vi "Host - Is FoE New.vi"(8 "error in (no error)":errorcluster, 10 "bitfile path in":path, 11 "Slave Ref in":refnum<k21>) -> (0 "error out":errorcluster, 3 "Slave Ref out":refnum<k21>)   [LabVIEW 2016, in "Scan Engine Custom Device.lvlib"]
uses:
  Scan Engine Custom Device.lvlib
  <resource>/objmgr/IndComECAT.rc
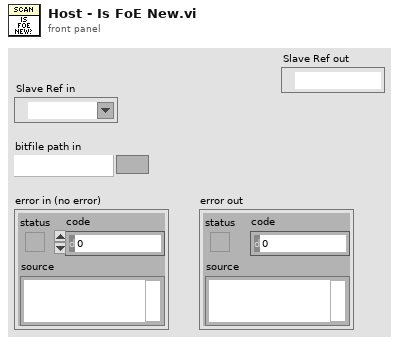
[diagram p1: front panel]
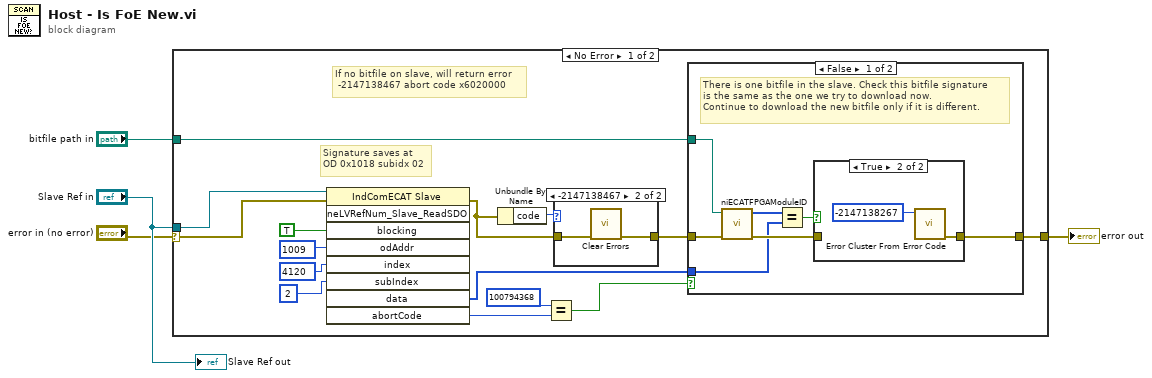
[diagram p0: block diagram]
diagram:
  n1 = case shown="No Error" "error in (no error)" {
    selector: "error in (no error)" -> [w14 w34]
    tunnel: "Slave Ref in" -> [w19 _]
    tunnel: "bitfile path in" -> [w18 _]
    tunnel: [w17 w34] -> w2
    frame No Error {
      # "Signature saves at \nOD 0x1018 subidx 02"
      # "If no bitfile on slave, will return error\n -2147138467 abort code x6020000"
      n2 = invoke class="IndComECAT Slave" method="neLVRefNum_Slave_ReadSDO"(reference=w19, error in=w14, "blocking"=TRUE, "odAddr"=u16 1009, "index"=u16 4120, "subIndex"=u8 2) -> (error out=w10:errorcluster, "data"=w13:u8[], "abortCode"=w11:u32)  [unwired: 3 in, 6 out]
      n3 = Unbundle By Name(w10) -> ("code"=w9:i32)
      n4 = Equal?(x=u32 100794368 ("Numeric 2"), y=w11) -> (x = y?=w15:bool)
      n5 = case shown="-2147138467" w9 {
        tunnel: w10 -> [w20 w22]
        tunnel: [w20 w21] -> w16
        frame 0, Default {
        }
        frame -2147138467 {
          n6 = call <vilib>:"Clear Errors.vi"("error in (no error)"=w22) -> ("error out"=w21:errorcluster)  [unwired: 5 in, 1 out]
        }
      }
      n7 = case shown="False" w15 {
        tunnel: w18 -> [w29 _]
        tunnel: w16 -> [w24 w33]
        tunnel: [w25 w33] -> w17
        tunnel: w13 -> [w23 _]
        frame False {
          # "There is one bitfile in the slave. Check this bitfile signature\nis the same as the one we try to download now.\nContinue to download the new bitfile only if it is different."
          n8 = call <vilib>:"niECATFPGAModuleID.vi"("error in"=w24, "Input bitfile path"=w29) -> ("error out"=w26:errorcluster, "Bitfile.SignatureRegister"=w27:u8[])  [unwired: 8 in]
          n9 = Equal?(x=w27, y=w23) -> (x = y?=w28:bool)
          n10 = case shown="True" w28 {
            tunnel: w26 -> [w30 _]
            tunnel: [w30 w31] -> w25
            frame False {
            }
            frame True {
              n11 = call <vilib>:"Error Cluster From Error Code.vi"("error code (0)"=-2147138267) -> ("error out"=w31:errorcluster)  [unwired: 8 in]
            }
          }
        }
        frame True {
        }
      }
    }
    frame Error {
    }
  }
  "error out" <- w2
  "Slave Ref out" <- "Slave Ref in"
